vi "Initialize.vi"(7 "Serial Configuration":T1={"Baud Rate"=57600, "Parity"=1, "Data Bits"=7, "Stop Bits"=10, "Flow Control"=0} {"Flow Control" items=["None", "XON/XOFF", "RTS/CTS", "XON/XOFF & RTS/CTS", "DTR/DSR", "XON/XOFF & DTR/DSR"]; "Stop Bits" items=["1.0"=10, "1.5"=15, "2.0"=20]; "Data Bits" items=["7"=7, "8"=8]; "Parity" items=["None", "Odd", "Even", "Mark", "Space"]; "Baud Rate" items=["300"=300, "600"=600, "1200"=1200, "2400"=2400, "4800"=4800, "9600"=9600, "19200"=19200, "38400"=38400, "57600"=57600]}, 8 "error in (no error)":errorcluster, 9 "Reset (True)":bool=TRUE, 10 "ID Query (True)":bool=TRUE, 11 "VISA resource name":refnum<visa-resource-name>) -> (0 "error out":errorcluster, 3 "VISA resource name out":refnum<visa-resource-name>)   [LabVIEW 2024, in "Lake Shore 336.lvlib"]
doc: "Establishes communication with the instrument and optionally performs an instrument identification query and/or an instrument reset. It also places the instrument in a default state needed for other instrument driver operations. Therefore, call this VI before calling other instrument driver VIs for this instrument. Generally, you need to call the <B>Initialize VI</B> only once at the beginning of an application."
uses:
  Lake Shore 336.lvlib
panel:
  # "(c) 2009 Lake Shore Cryotronics Inc.  ALL RIGHTS RESERVED."
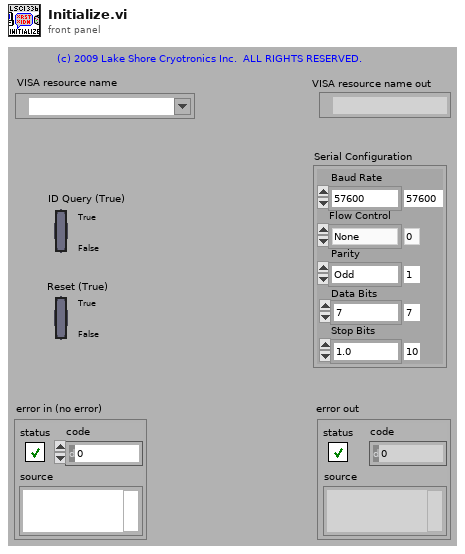
[diagram p1: front panel]
types:
  T1 = cluster{"Baud Rate":u32, "Parity":u16, "Data Bits":u16, "Stop Bits":u16, "Flow Control":u16}
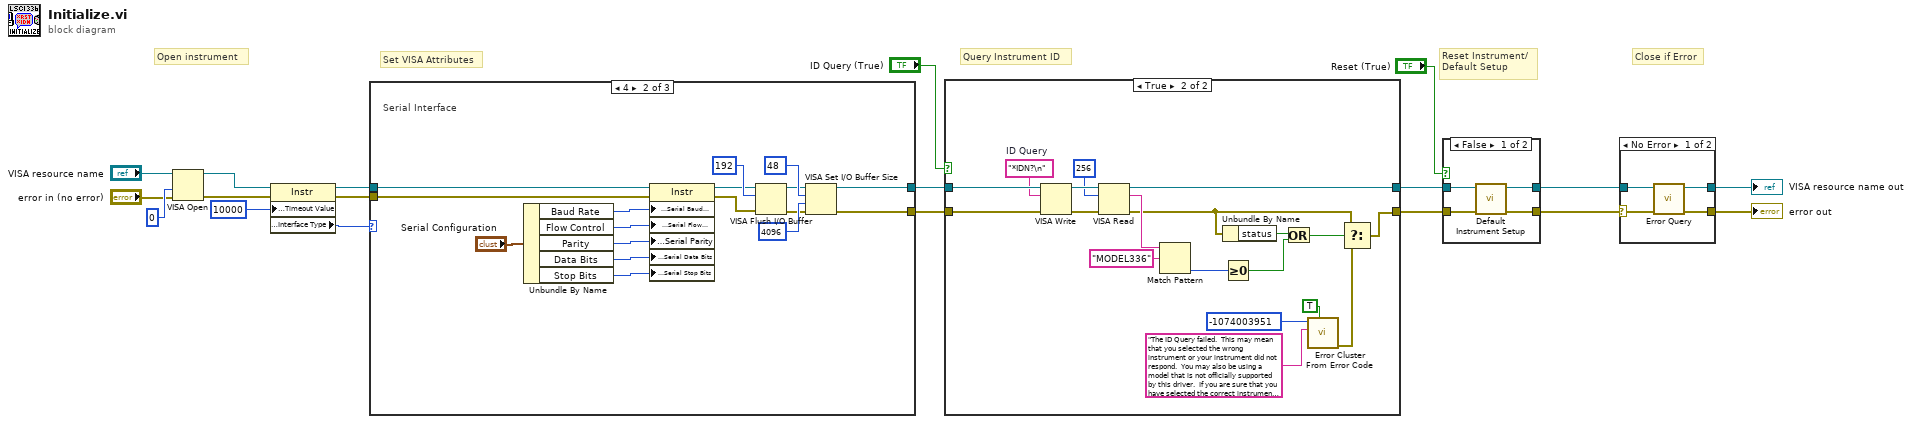
[diagram p0: block diagram]
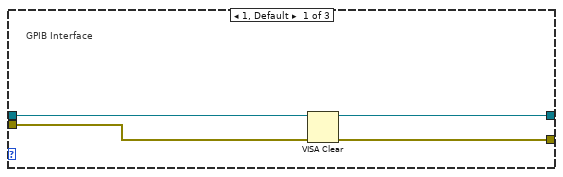
[diagram p2: hidden frame]
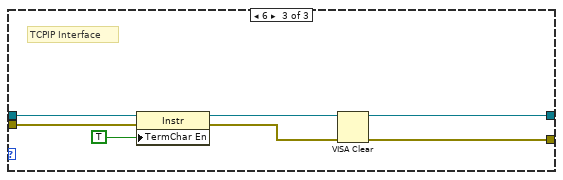
[diagram p3: hidden frame]
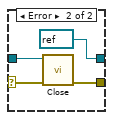
[diagram p4: hidden frame]
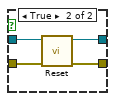
[diagram p5: hidden frame]
diagram:
  # "Set VISA Attributes"
  # "Close if Error"
  # "Query Instrument ID"
  # "Reset Instrument/\nDefault Setup"
  # "Open instrument"
  n1 = VISA Open(access mode=u32 0, error in (no error)="error in (no error)", VISA resource name="VISA resource name") -> (VISA resource name=w9:refnum<visa-resource-name>, error out=w8:errorcluster)  [unwired: 2 in]
  n2 = property class="Instr"(reference=w9, error in=w8, "General Settings:Timeout Value"=u32 10000) -> (reference out=w7:refnum<visa-resource-name>, error out=w6:errorcluster, "Interface Information:Interface Type"=w5:u16)
  n3 = case shown="4" w5 {
    tunnel: [w23 w27 w43] -> w2
    tunnel: [w22 w26 w41] -> w1
    tunnel: w7 -> [w20 w24 w47]
    tunnel: w6 -> [w21 w25 w46]
    frame 1, Default {
      # "GPIB Interface"
      n4 = VISA Clear(VISA resource name=w20, error in (no error)=w21) -> (VISA resource name out=w23:refnum<visa-resource-name>, error out=w22:errorcluster)
    }
    frame 4 {
      # "Serial Interface"
      n5 = Unbundle By Name("Serial Configuration") -> ("Baud Rate"=w35:u32, "Flow Control"=w39:u16, "Parity"=w37:u16, "Data Bits"=w36:u16, "Stop Bits"=w40:u16)
      n6 = property class="Instr"(reference=w24, error in=w25, "Serial Settings:Serial Baud Rate"=w35, "Serial Settings:Serial Flow Control"=w39, "Serial Settings:Serial Parity"=w37, "Serial Settings:Serial Data Bits"=w36, "Serial Settings:Serial Stop Bits"=w40) -> (reference out=w31:refnum<visa-resource-name>, error out=w29:errorcluster)
      n7 = VISA Flush I/O Buffer(VISA resource name=w31, mask (16)=u16 192, error in (no error)=w29) -> (VISA resource name out=w28:refnum<visa-resource-name>, error out=w30:errorcluster)
      n8 = VISA Set I/O Buffer Size(VISA resource name=w28, mask (16)=u16 48, size (4096)=u32 4096 ("size (0)"), error in (no error)=w30) -> (VISA resource name out=w27:refnum<visa-resource-name>, error out=w26:errorcluster)
    }
    frame 6 {
      # "TCPIP Interface"
      n9 = property class="Instr"(reference=w47, error in=w46, "TermChar En"=TRUE) -> (reference out=w44:refnum<visa-resource-name>, error out=w42:errorcluster)
      n10 = VISA Clear(VISA resource name=w44, error in (no error)=w42) -> (VISA resource name out=w43:refnum<visa-resource-name>, error out=w41:errorcluster)
    }
  }
  n11 = case shown="True" "ID Query (True)" {
    tunnel: [w48 w68] -> w18
    tunnel: [w49 w51] -> w19
    tunnel: w2 -> [w49 w66]
    tunnel: w1 -> [w48 w67]
    frame False {
    }
    frame True {
      w52 = "*IDN?\n"  # ID Query
      n12 = VISA Write(VISA resource name=w66, write buffer=w52, error in (no error)=w67) -> (VISA resource name out=w64:refnum<visa-resource-name>, error out=w63:errorcluster)  [unwired: 1 out]
      n13 = VISA Read(VISA resource name=w64, byte count=u32 256, error in (no error)=w63) -> (VISA resource name out=w51:refnum<visa-resource-name>, read buffer=w65:string, error out=w50:errorcluster)  [unwired: 1 out]
      n14 = Match Pattern(string=w65, regular expression="MODEL336") -> (offset past match=w56:i32)  [unwired: 1 in, 3 out]
      n15 = Unbundle By Name(w50) -> ("status"=w55:bool)
      n16 = Greater Or Equal To 0?(x=w56) -> (x >= 0?=w53:bool)
      n17 = Or(x=w55, y=w53) -> (x .or. y?=w54:bool)
      n18 = call <vilib>:"Error Cluster From Error Code.vi"("show call chain? (False)"=TRUE, "error message (\"\")"="The ID Query failed.  This may mean that you selected the wrong instrument or your instrument did not respond.  You may also be using a model that is not officially supported by this driver.  If you are sure that you have selected the correct instrument and it is responding, try disabling the ID Query." ("Source (VI Name)"), "error code (0)"=-1074003951 ("Code")) -> ("error out"=w60:errorcluster)  [unwired: 6 in]
      n19 = Select(t=w50, s=w54, f=w60) -> (s? t:f=w68:errorcluster)
    }
  }
  n20 = case shown="False" "Reset (True)" {
    tunnel: w18 -> [w71 w73]
    tunnel: [w70 w76] -> w12
    tunnel: w19 -> [w72 w74]
    tunnel: [w69 w75] -> w13
    frame False {
      n21 = call "Default Instrument Setup.vi"("error in (no error)"=w71, "VISA resource name"=w72) -> ("error out"=w70:errorcluster, "VISA resource name out"=w69:refnum<visa-resource-name>)  [unwired: 8 in]
    }
    frame True {
      n22 = call "Reset.vi"("error in (no error)"=w73, "VISA resource name"=w74) -> ("error out"=w76:errorcluster, "VISA resource name out"=w75:refnum<visa-resource-name>)  [unwired: 8 in]
    }
  }
  n23 = case shown="No Error" w12 {
    selector: w12 -> [w80 w82]
    tunnel: w13 -> [w79 w83]
    tunnel: [w78 refnum<visa-resource-name> refnum ("VISA resource name out")] -> w15
    tunnel: [w77 w84] -> w14
    frame No Error {
      n24 = call "Error Query.vi"("error in (no error)"=w80, "VISA resource name"=w79) -> ("error out"=w77:errorcluster, "VISA resource name out"=w78:refnum<visa-resource-name>)  [unwired: 7 in, 1 out]
    }
    frame Error {
      n25 = call "Close.vi"("error in (no error)"=w82, "VISA resource name"=w83) -> ("error out"=w84:errorcluster)  [unwired: 9 in]
    }
  }
  "VISA resource name out" <- w15
  "error out" <- w14
